vi "E5.vi"() -> ()   [LabVIEW 2018]
panel:
  out "XY Graph":cluster{"X":dbl, "Y":dbl}[](graph)
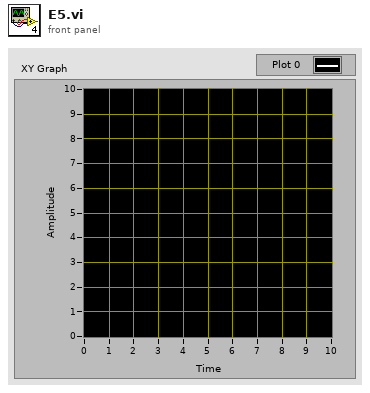
[diagram p1: front panel]
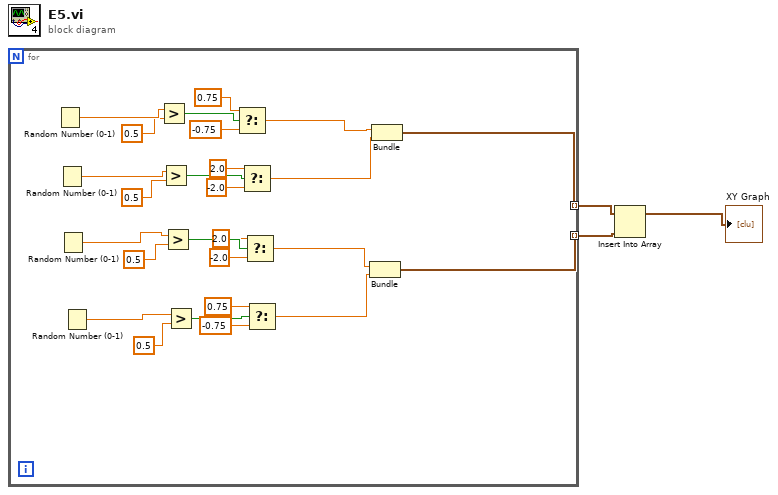
[diagram p0: block diagram]
diagram:
  n1 = for {
    tunnel: [w5] -> w3 mode=indexing
    tunnel: [w4] -> w2 mode=indexing
    n2 = Random Number (0-1)() -> (number: 0 to 1=w29:dbl)
    n3 = Random Number (0-1)() -> (number: 0 to 1=w28:dbl)
    n4 = Random Number (0-1)() -> (number: 0 to 1=w27:dbl)
    n5 = Random Number (0-1)() -> (number: 0 to 1=w26:dbl)
    n6 = Greater?(x=w29, y=0.5) -> (0:w21:bool)
    n7 = Greater?(x=w28, y=0.5) -> (0:w20:bool)
    n8 = Greater?(x=w27, y=0.5) -> (0:w19:bool)
    n9 = Greater?(x=w26, y=0.5) -> (0:w18:bool)
    n10 = Select(t=0.75, s=w21, f=-0.75) -> (s? t:f=w9:dbl)
    n11 = Select(t=2.0, s=w20, f=-2.0) -> (s? t:f=w8:dbl)
    n12 = Select(t=2.0, s=w19, f=-2.0) -> (s? t:f=w7:dbl)
    n13 = Select(t=0.75, s=w18, f=-0.75) -> (s? t:f=w6:dbl)
    n14 = Bundle("f"=w7, "f"=w6) -> (w5:cluster{"f":dbl, "f":dbl})  [unwired: 1 in]
    n15 = Bundle("f"=w9, "f"=w8) -> (w4:cluster{"f":dbl, "f":dbl})  [unwired: 1 in]
  }
  n16 = Insert Into Array(array=w2, new element=w3) -> (→"XY Graph":cluster{"f":dbl, "f":dbl}[])  [unwired: 1 in]
